vi "Modbus_Slave.vi"() -> ()   [LabVIEW 2020]
uses:
  <vilib>/NI/Modbus Library/Data Model/Device Data Model.lvclass
  <vilib>/NI/Modbus Library/API/Wrapper/Create TCP Slave.vi
  <vilib>/ErrorRing/Error Ring.xnode
  <vilib>/NI/Modbus Library/API/Slave/Modbus Slave.lvclass
  <vilib>/NI/Modbus Library/API/Wrapper/API Main.lvlib
panel:
  out "Array 2":u16[](array[slide]) scale=0.0..100.0
  in  "stop":bool
  out "Array":bool[](array[boolean])
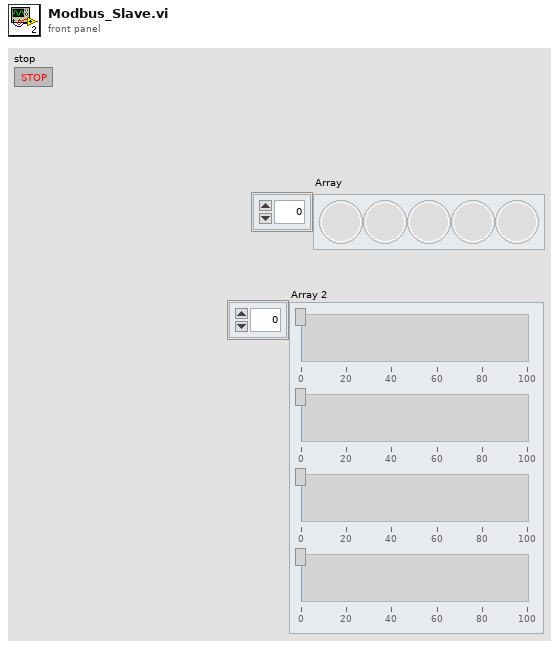
[diagram p1: front panel]
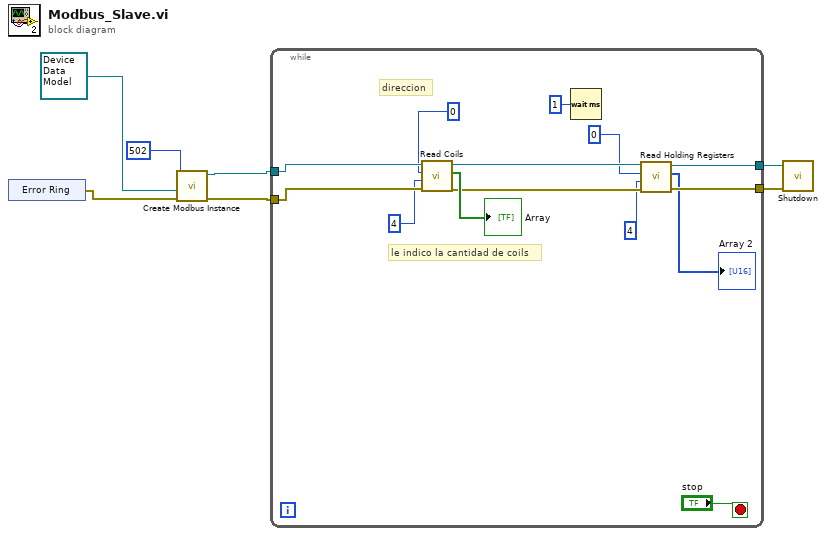
[diagram p0: block diagram]
diagram:
  n1 = xnode "Error Ring"() -> ("error out"=w5:errorcluster)
  n2 = call-poly <vilib>:"Create Modbus Instance.vi"("error in"=w5, "device data model"=refnum<class "Device Data Model.lvclass"> refnum, "port (502)"=u16 502) -> ("error out"=w3:errorcluster, "TCP slave instance"=w4:refnum<class "Modbus Slave.lvclass">)  [unwired: 7 in]
  n3 = while {
    tunnel: w4 -> [w21]
    tunnel: w3 -> [w20]
    tunnel: [w13] -> w2
    tunnel: [w12] -> w1
    stop <- "stop" stop-if-true
    # "direccion"
    # "le indico la cantidad de coils"
    n4 = call-dynamic "Read Coils.vi"("error in"=w20, "number of inputs"=u16 4, "starting address"=u16 0, "Modbus slave in"=w21) -> ("error out"=w11:errorcluster, "coils"=→"Array":bool[], "Modbus slave out"=w14:refnum<class "Modbus Slave.lvclass">)  [unwired: 5 in]
    n5 = Wait (ms)(milliseconds to wait=u32 1) -> ()  [unwired: 1 out]
    n6 = call-dynamic "Read Holding Registers.vi"("error in"=w11, "number of inputs"=u16 4, "starting address"=u16 0, "Modbus slave in"=w14) -> ("error out"=w12:errorcluster, "register values"=→"Array 2":u16[], "Modbus slave out"=w13:refnum<class "Modbus Slave.lvclass">)  [unwired: 5 in]
  }
  n7 = call-dynamic "Shutdown.vi"("error in"=w1, "Modbus slave in"=w2) -> ()  [unwired: 9 in, 1 out]
